vi "gg0.vi"(1 "B":dbl, 2 "A":dbl) -> (0 "C":dbl)   [LabVIEW 2020]
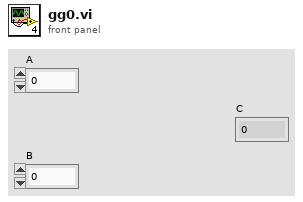
[diagram p1: front panel]
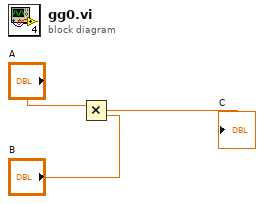
[diagram p0: block diagram]
diagram:
  n1 = Multiply(x="A", y="B") -> (x*y=→"C":dbl)
